vi "Path_To_Pose_Eng.vi"(11 "Path Sample":T4) -> (3 "out POSe":T1)   [LabVIEW 2019, in "PathExecution_Library.lvlib"]
uses:
  PathExecution_Library.lvlib
  PATH_SAMPLE.ctl
  POSE.ctl
  TRANSLATION.ctl
  ROTATION.ctl
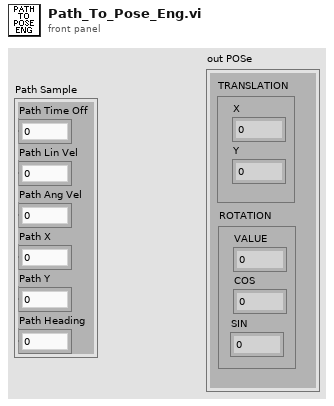
[diagram p1: front panel]
types:
  T1 = typedef "PathExecution_Library.lvlib/POSE.ctl" = cluster{"TRANSLATION":T2, "ROTATION":T3}
  T2 = typedef "PathExecution_Library.lvlib/TRANSLATION.ctl" = cluster{"X":dbl, "Y":dbl}
  T3 = typedef "PathExecution_Library.lvlib/ROTATION.ctl" = cluster{"VALUE":dbl, "COS":dbl, "SIN":dbl}
  T4 = typedef "PathExecution_Library.lvlib/PATH_SAMPLE.ctl" = cluster{"Path Lin Vel":dbl, "Path Ang Vel":dbl, "Path X":dbl, "Path Y":dbl, "Path Heading":dbl, "Path Time Off":dbl}
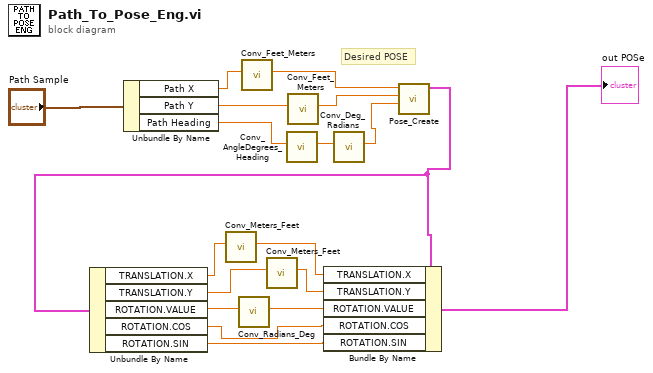
[diagram p0: block diagram]
diagram:
  # "Desired POSE"
  n1 = Unbundle By Name("Path Sample") -> ("Path X"=w15:dbl, "Path Y"=w17:dbl, "Path Heading"=w13:dbl)
  n2 = call "Conv_Feet_Meters.vi"("Feet"=w15) -> ("Meters"=w16:dbl)  [unwired: 10 in]
  n3 = call "Conv_AngleDegrees_Heading.vi"("Degrees"=w13) -> ("Radians"=w2:dbl)  [unwired: 10 in]
  n4 = call "Conv_Feet_Meters.vi"("Feet"=w17) -> ("Meters"=w18:dbl)  [unwired: 10 in]
  n5 = call "Conv_Deg_Radians.vi"("Degress"=w2) -> ("Radians"=w1:dbl)  [unwired: 10 in]
  n6 = call "Pose_Create.vi"("Heading"=w1, "Y"=w18, "X"=w16) -> ("out POSe"=w3:T1)  [unwired: 8 in]
  n7 = Unbundle By Name(w3) -> ("TRANSLATION.X"=w11:dbl, "TRANSLATION.Y"=w10:dbl, "ROTATION.VALUE"=w12:dbl, "ROTATION.COS"=w8:dbl, "ROTATION.SIN"=w7:dbl)
  n8 = call "Conv_Meters_Feet.vi"("Meters"=w11) -> ("Feet"=w5:dbl)  [unwired: 10 in]
  n9 = call "Conv_Radians_Deg.vi"("Radians"=w12) -> ("Degrees"=w9:dbl)  [unwired: 10 in]
  n10 = call "Conv_Meters_Feet.vi"("Meters"=w10) -> ("Feet"=w6:dbl)  [unwired: 10 in]
  n11 = Bundle By Name(cluster=w3, "TRANSLATION.X"=w5, "TRANSLATION.Y"=w6, "ROTATION.VALUE"=w9, "ROTATION.COS"=w8, "ROTATION.SIN"=w7) -> (→"out POSe":T1)
